vi "plot_data.vi"(8 "error in (no error)":errorcluster, 10 "panel.lvclass":refnum<class "panel.lvclass">, 11 "data in":refnum<class "data.lvclass">) -> (0 "error out":errorcluster, 3 "data out":refnum<class "data.lvclass">)   [LabVIEW 2015, in "data.lvclass"]
uses:
  data.lvclass
  UI/panel_class/panel.lvclass
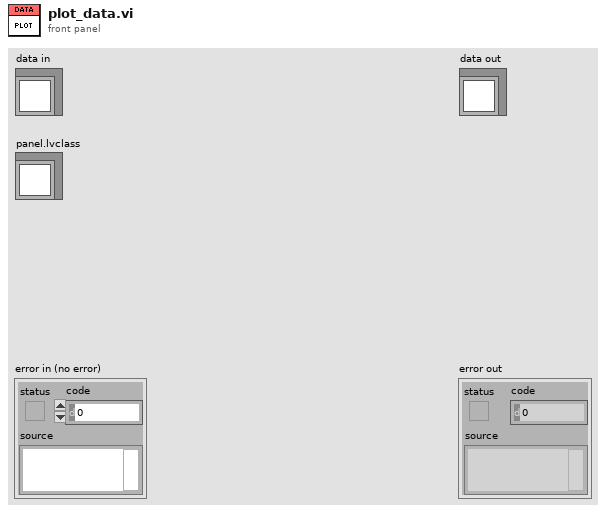
[diagram p1: front panel]
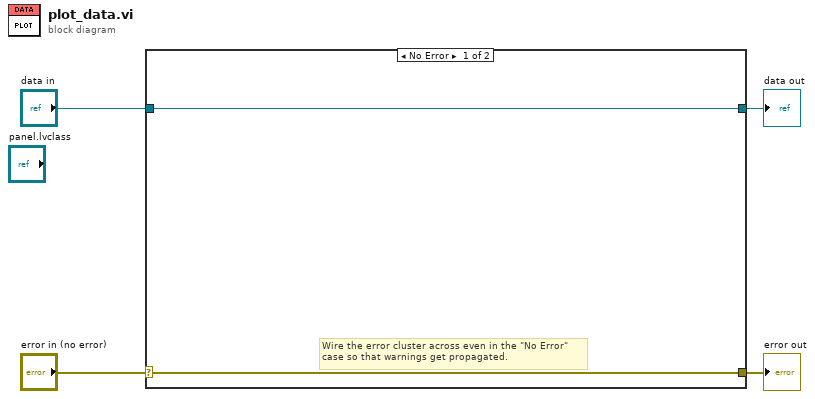
[diagram p0: block diagram]
diagram:
  n1 = case shown="No Error" "error in (no error)" {
    selector: "error in (no error)" -> [w5 w8]
    tunnel: [w5 w8] -> w3
    tunnel: [w6 w7] -> w1
    tunnel: "data in" -> [w6 w7]
    frame No Error {
      # "Wire the error cluster across even in the \"No Error\"\ncase so that warnings get propagated."
    }
    frame Error {
    }
  }
  "error out" <- w3
  "data out" <- w1
